vi "Write Diode Log.vi"(4 "TLUP_Temperatures":waveform(dbl)[](array[waveform]), 5 "TED":waveform(dbl)[](array[waveform]), 6 "TVC_Temperatures":waveform(dbl)[](array[waveform]), 7 "Diode Currents":waveform(dbl)[](array[waveform]), 10 "LogFile path":path) -> ()   [LabVIEW 2025]
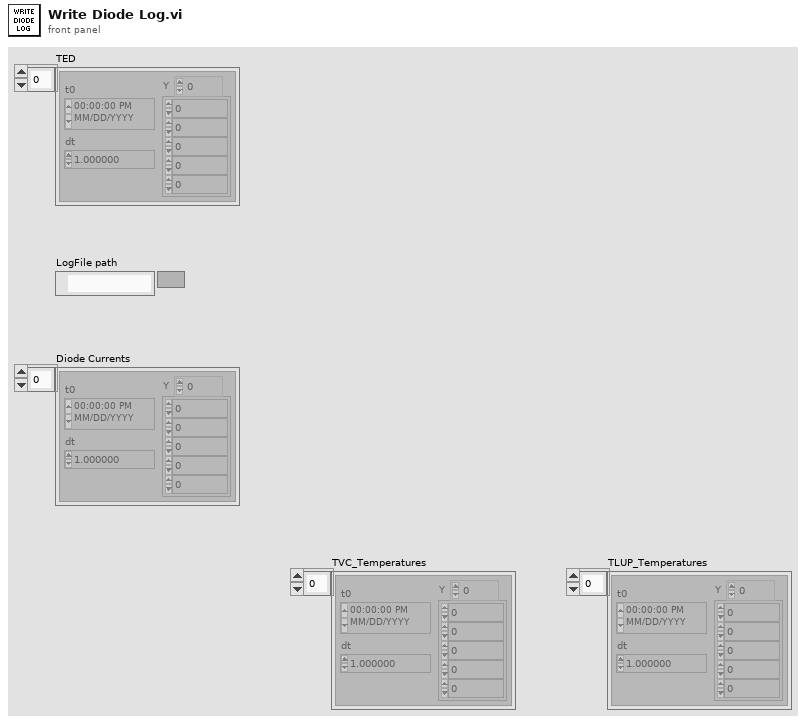
[diagram p1: front panel]
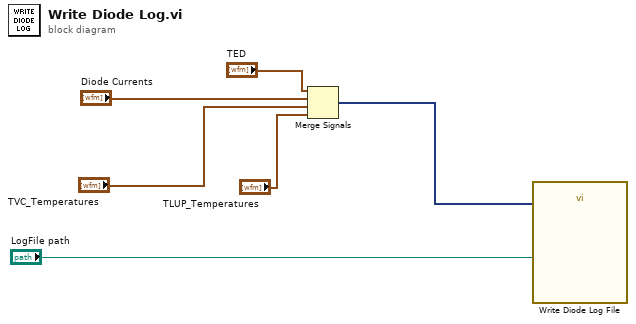
[diagram p0: block diagram]
diagram:
  n1 = Merge Signals("TED", "Diode Currents", "TVC_Temperatures", "TLUP_Temperatures") -> (w3:dynamicdata)
  n2 = call "Write Diode Log File"("Signals"=w3, "Filename"="LogFile path") -> ()  [unwired: 15 in, 3 out]
